vi "Set Array of TA Binding.vi"(8 "error in (no error)":errorcluster, 10 "Array of TA Binding":T1[](array[typedef]), 11 "Motions Configuration in":refnum<class "Motions Configuration.lvclass">) -> (0 "error out":errorcluster, 3 "Motions Configuration out":refnum<class "Motions Configuration.lvclass">)   [LabVIEW 2016, in "Hardware.lvlib" / "Motions.lvlib" / "Motions Configuration.lvclass"]
uses:
  <userlib>/Common Components/Hardware/Abstract System/Motions/Motions Config/Motions Configuration.lvclass
  <userlib>/Common Components/Hardware/Abstract System/Motions/Motions/TA Binding Data.ctl
  <userlib>/Common Components/Hardware/Abstract System/Motions/Motions Config/Motions Configuration.lvclass/Motions Configuration.ctl
  <userlib>/Common Components/Hardware/Abstract System/Motions/Motions/Motions.lvclass/Motions.ctl
  <userlib>/Common Components/Hardware/Abstract System/Motions/Motions/Motions.lvclass
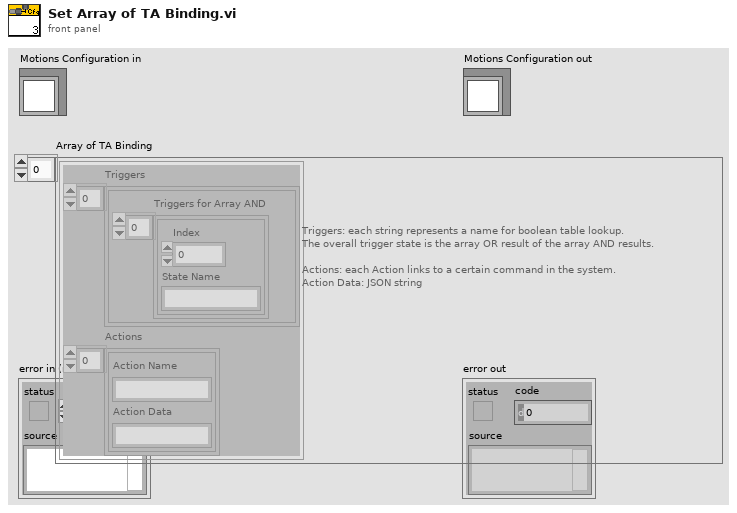
[diagram p1: front panel]
types:
  T1 = typedef "Hardware.lvlib/Motions.lvlib/Motions.lvclass/TA Binding Data.ctl" = cluster{"Triggers":cluster{"Triggers for Array AND":cluster{"Index":u8, "State Name":string}[]}[], "Actions":cluster{"Action Name":string, "Action Data":string}[]}
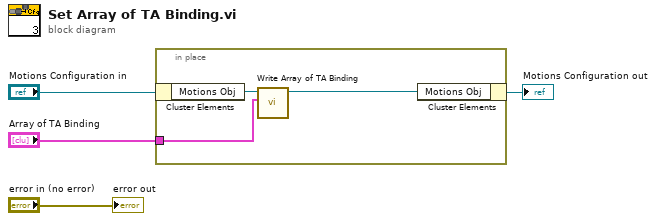
[diagram p0: block diagram]
diagram:
  n1 = in-place {
    in-place-border: "Array of TA Binding" -> [w5]
    n2 = in-place-cluster #1("Motions Configuration in") -> ("Motions Obj"=w7:refnum<class "Motions.lvclass">)
    n3 = call <userlib>:"Write Array of TA Binding.vi"("Array of TA Binding"=w5, "Motions in"=w7) -> ("Motions out"=w6:refnum<class "Motions.lvclass">)  [unwired: 9 in]
    n4 = in-place-cluster #1("Motions Obj"=w6) -> (→"Motions Configuration out":refnum<class "Motions Configuration.lvclass">)
  }
  "error out" <- "error in (no error)"
